vi "Init Data Object.vi"(11 "xData in":refnum<class "xData.lvclass">) -> (3 "xData out":refnum<class "xData.lvclass">)   [LabVIEW 2014, in "xData.lvclass"]
uses:
  xData.lvclass
  reusable/Data/Data.lvclass
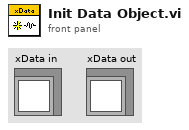
[diagram p1: front panel]
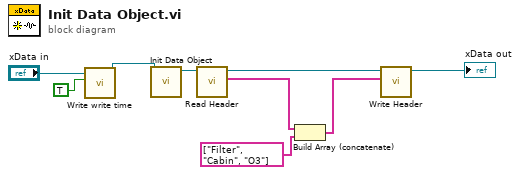
[diagram p0: block diagram]
diagram:
  n1 = call "Write write time.vi"("write time"=TRUE, "Data in"="xData in") -> ("Data out"=w8:refnum<class "xData.lvclass">)  [unwired: 8 in, 1 out]
  n2 = call-parent "Init Data Object.vi"("Data in"=w8) -> ("Data out"=w6:refnum<class "xData.lvclass">)  [unwired: 10 in]
  n3 = call "Read Header.vi"("Data in"=w6) -> ("Header"=w5:string[], "Data out"=w2:refnum<class "xData.lvclass">)  [unwired: 8 in, 1 out]
  n4 = Build Array (concatenate)(w5, string[] ["Filter", "Cabin", "O3"] ("Header")) -> (w3:string[])
  n5 = call "Write Header.vi"("Header"=w3, "Data in"=w2) -> ("Data out"=→"xData out":refnum<class "xData.lvclass">)  [unwired: 8 in, 1 out]
